vi "选择某框-子界面.vi"() -> ()   [LabVIEW 2018]
uses:
  <vilib>/vision/NI_Vision_Development_Module.lvlib
  <vilib>/Utility/NIReport.llb/Report Type.ctl
  <vilib>/Utility/NIReport.llb/NI_ReportGenerationCore.lvlib
panel:
  out "框组":T1(array[cluster])
  out "框号":dbl format="%#_13g"
  out "选中框灰度表":u32[](graph)
  out "最小灰度值":sgl
  out "最大灰度值":sgl
  out "平均值":sgl
  out "标准差":sgl
  in  "条件1-面积判断":T3(array[cluster]) {"Measurement Parameter" items=["Area"]; "下限" format="%.2f"; "上限" format="%.2f"}
  out "显示结果":string caption="所选区域信息"
  out "Particle Measurements (Pixels)":dbl[][](array[numeric]) format="%.2f"
  in  "报告生成":bool
  out "检查文件路径是否正确":bool caption="文件或文件夹存在？"
  out "保存路径":path
  in  "产品序号":string
  in  "部位":string="位置1"
  in  "类型":string="类型1"
  in  "合格性":string="合格"
  in  "检验人":string
  out "模板路径":path
  in  "分隔符（'\\'代码显示）":string="\t"
  in  "格式字符串":string="%f"
  out "所选区域检测结果":string[][](table)
  in  "查看完毕":bool
  in  "Color":u32[](array[colorbox])=[3381759, 16776770, 16777225, 6618880]
  in  "Overlay Type":u16[](array[ring])=[2, 1, 3, 0] items=["Rectangle", "Numbers", "Points", "Lines"]
  in  "条件2-灰度阈值":cluster{"下限":sgl, "上限":sgl}={"下限"=128.0, "上限"=255.0} {"下限" min=0 max=255 step=1; "上限" min=0 max=255 step=1}
  in  "Tab Control":T4
  out "原图":T5(plugin-control) caption="Original Image"
  out "阈值处理":T5(plugin-control) caption="Threshold Image"
  out "面积筛选":T5(plugin-control) caption="Reject Border and Fill Holes"
  out "缺陷统计":T5(plugin-control) caption="Filter Out Non Circles and Overlay Particle Area"
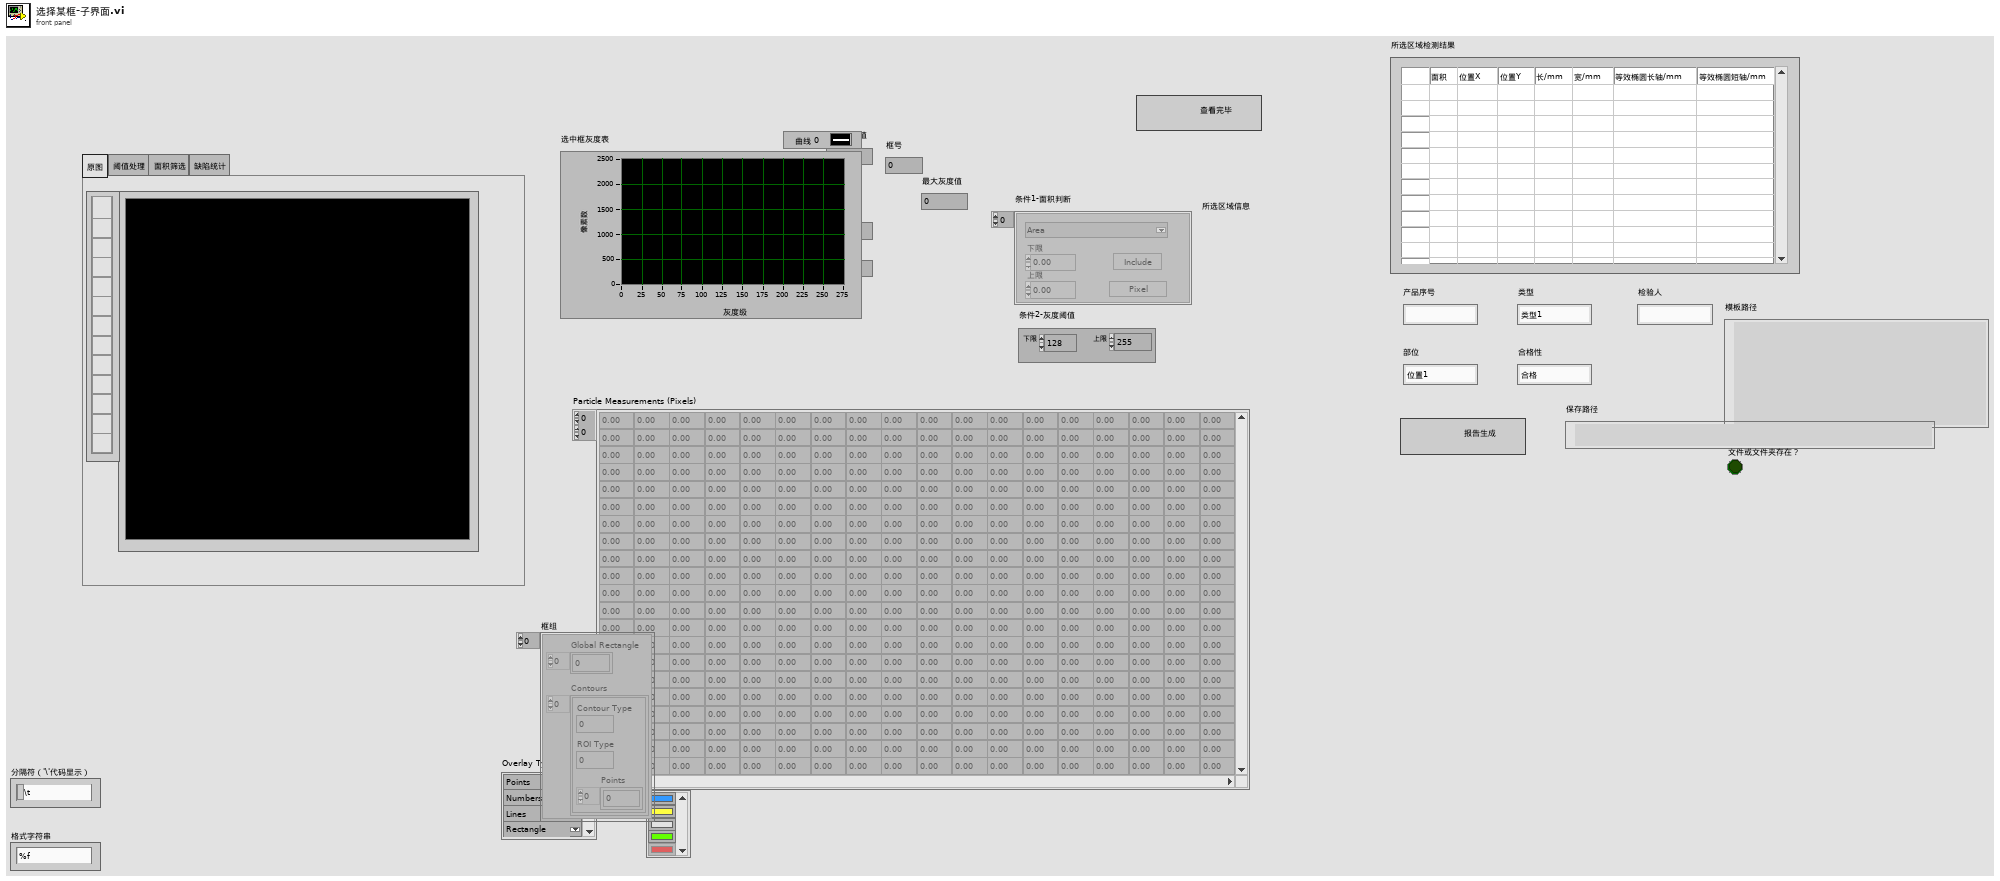
[diagram p1: front panel]
types:
  T1 = cluster{"Global Rectangle":i32[], "Contours":cluster{"Contour Type":u32, "ROI Type":u32, "Points":i32[]}[]}[]
  T2 = typedef "Particle Parameters" = i32
  T3 = cluster{"Measurement Parameter":T2, "下限":dbl, "上限":dbl, "Range":bool, "Measurement Type":bool}[]
  T4 = typedef "控件 1.ctl" = enum32{"原图", "阈值处理", "面积筛选", "缺陷统计"}
  T5 = typedef "IMAQ Image.ctl" = refnum<image>
  T6 = typedef "NI_ReportGenerationCore.lvlib/Report Type.ctl" = enum16{"HTML", "Word", "Excel"}
  T7 = cluster{"position (excel)":cluster{"row":i32, "column":i32}, "name (excel)":string, "bookmark (word)":string}
  T8 = typedef "Image Type" = u32
  T9 = cluster{"Global Rectangle":i32[], "Contours":cluster{"Contour Type":u32, "ROI Type":u32, "Points":i32[]}[]}
  T10 = typedef "IMAQ Rectangle" = cluster{"Left":i32, "Top":i32, "Right":i32, "Bottom":i32, "Rotation":dbl}
  T11 = cluster{"条件2-灰度阈值":cluster{"下限":sgl, "上限":sgl}, "Pixel Measurements":T2[], "Overlay Type":u16[], "Color":u32[]}
  T12 = cluster{"histogram":u32[], "Minimal Value":sgl, "Maximal Value":sgl, "Starting Value":sgl, "Interval Width":sgl, "Mean Value":sgl, "Standard  Variation":sgl, "Area (pixels)":i32}
  T13 = cluster{"Desired Font (Application)":enum16{"User-specified Font", "Application Font", "System Font", "Dialog Font"}, "[User-specified Font]":cluster{"Font Name":string, "Size":i16, "Strikeout?":bool, "Italic?":bool, "Underline?":bool, "Outline?":bool, "Shadow?":bool, "Bold?":bool, "Rotation Angle":dbl}, "Horizontal Alignment":i16, "Vertical Alignment":i16}
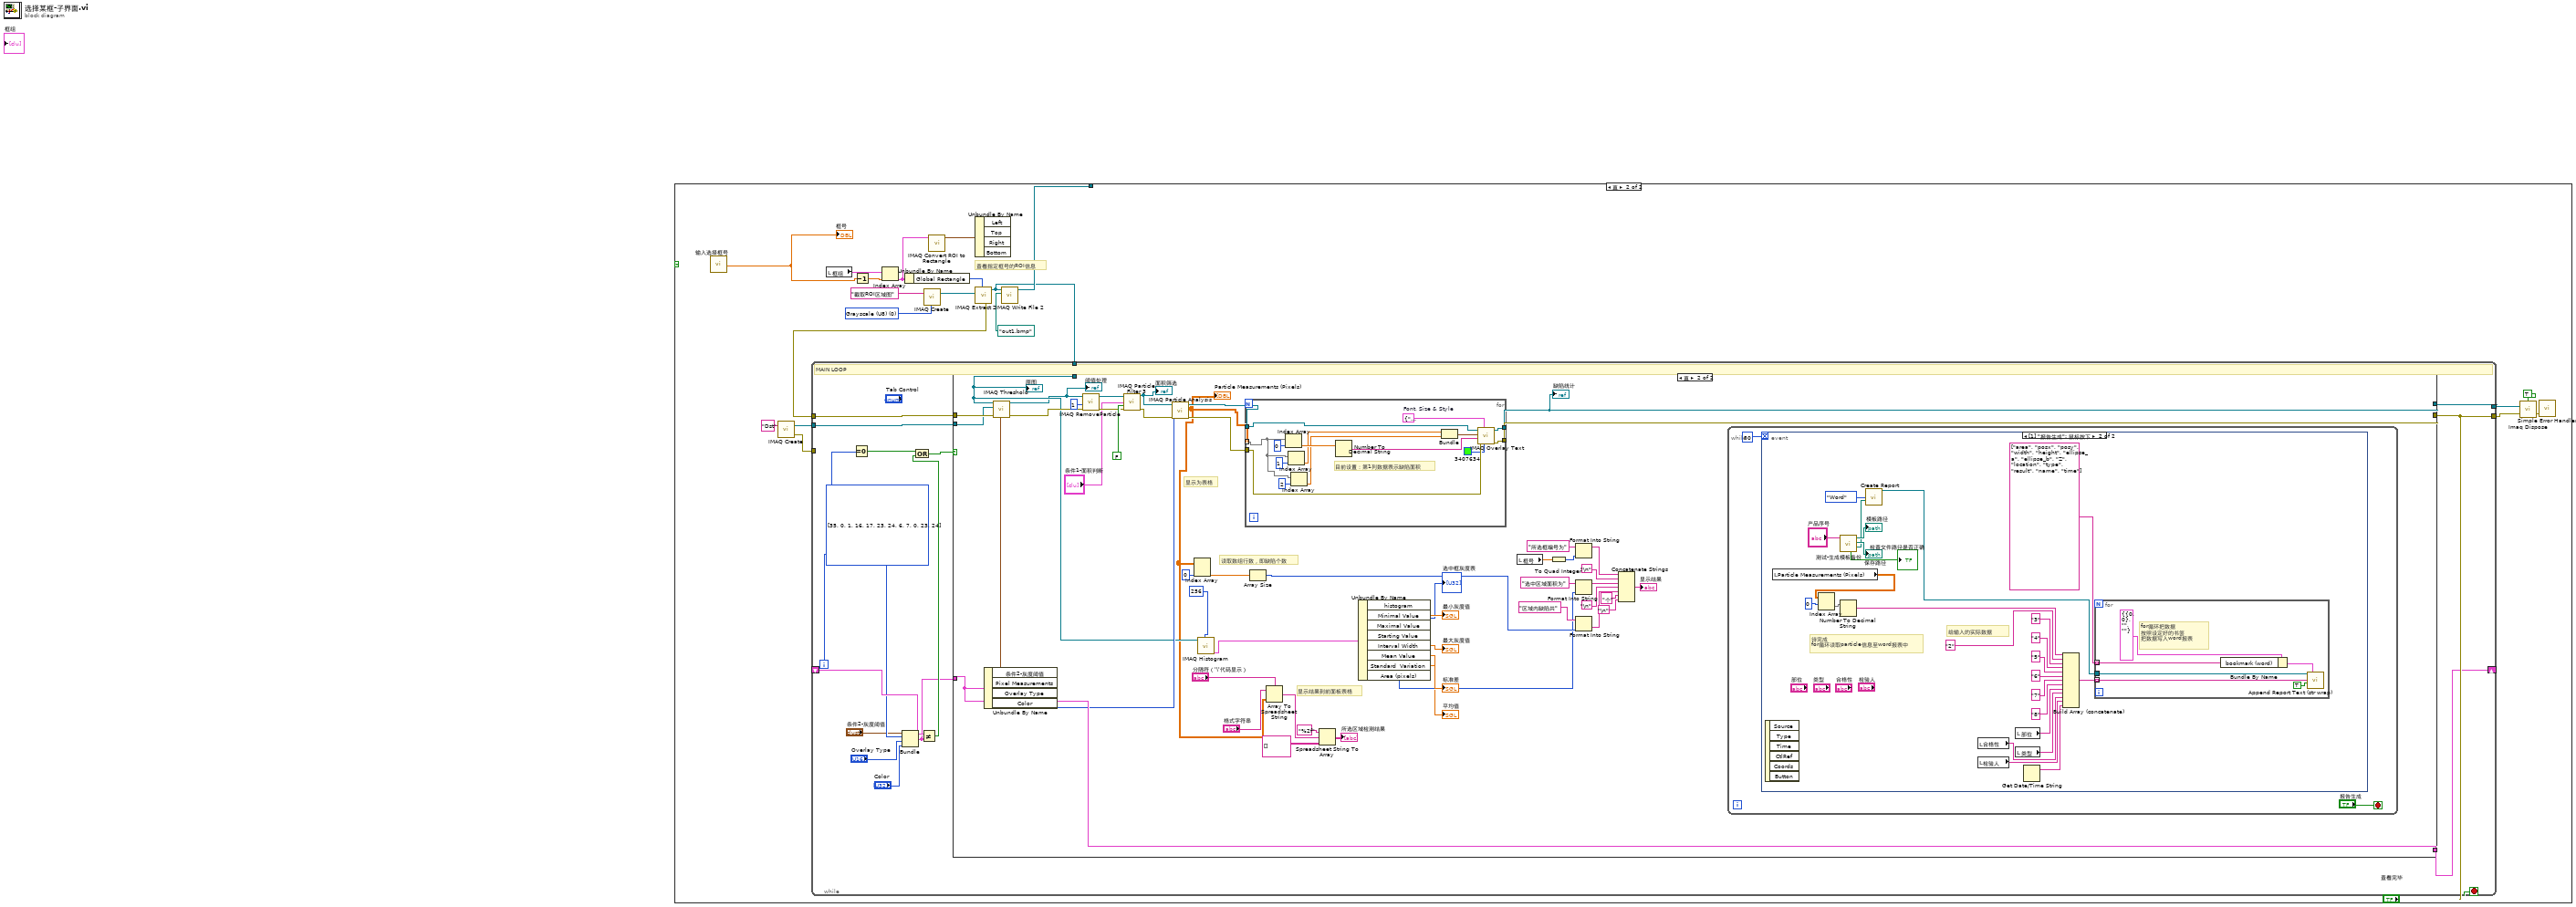
[diagram p0: block diagram]
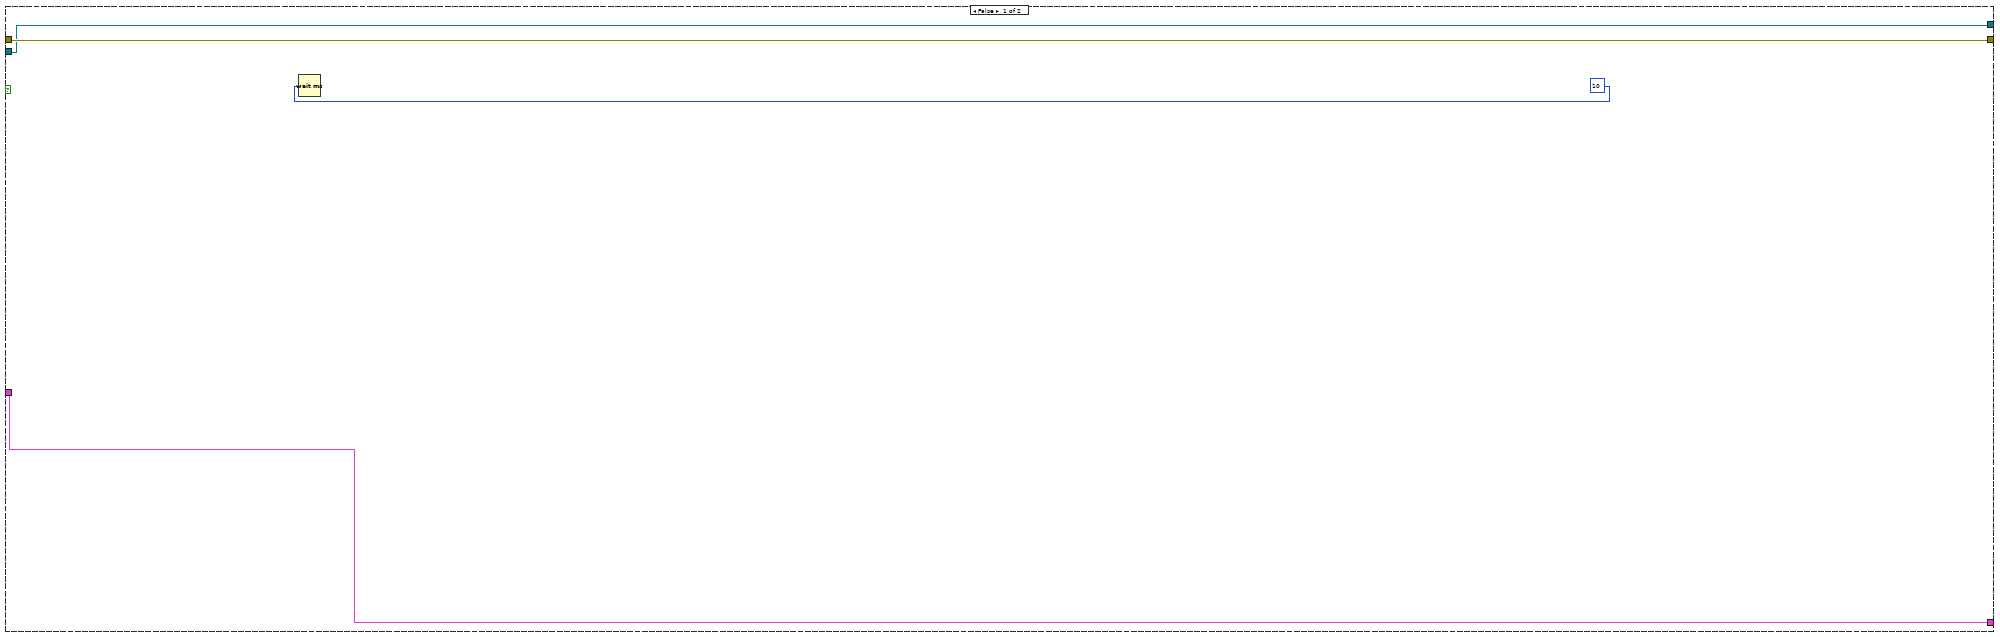
[diagram p3: hidden frame]
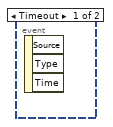
[diagram p4: hidden frame]
diagram:
  n1 = case shown="真" {
    selector: _ -> [_ _]
    tunnel: _ -> [_ w13]
    frame False {
      # "用户取消操作"
    }
    frame True {
      w17 = T8 0 items=["Grayscale (U8)", "Grayscale (I16)", "Grayscale (SGL)", "Complex (CSG)", "RGB (U32)", "HSL (U32)", "RGB (U64)", "Grayscale (U16)"] ("Image Type")
      # "查看指定框号的ROI信息"
      n2 = call "输入选择框号"() -> ("框号"=w1:dbl)  [unwired: 17 in, 2 out]
      "框号" <- w1
      n3 = call "IMAQ Create"("Image Name"="Dst") -> ("New Image"=w6:T5, "error out"=w5:errorcluster)  [unwired: 4 in]
      n4 = local read "框组"() -> (w19:T1)
      n5 = Decrement(x=w1) -> (x-1=w20:dbl)
      n6 = Index Array(array=w19, index=w20) -> (element=w12:T9)
      n7 = Unbundle By Name(w12) -> ("Global Rectangle"=w18:i32[])
      n8 = call "IMAQ Create"("Image Name"="截取ROI区域图", "Image Type"=w17) -> ("New Image"=w15:T5)  [unwired: 3 in, 1 out]
      n9 = call "IMAQ Convert ROI to Rectangle"("ROI Descriptor"=w12) -> ("Rectangle"=w14:T10)  [unwired: 8 in, 1 out]
      n10 = Unbundle By Name(w14) -> ()  [unwired: 4 out]
      n11 = call "IMAQ Extract 2"("Optional Rectangle"=w18, "Image Dst"=w15, "Image Src"=w13) -> ("error out"=w3:errorcluster, "Image Dst Out"=w2:T5)  [unwired: 7 in]
      n12 = while "MAIN LOOP" {
        tunnel: w3 -> [w28]
        tunnel: [w37] -> w10
        shift-right: [w34] -> _
        shift-left: _ -> [w32]
        tunnel: w6 -> [w29]
        tunnel: w5 -> [_]
        tunnel: [w27] -> w4
        tunnel: w2 -> [w24]
        i -> [w36]
        stop <- w38 stop-if-true
        w26 = T2[] [35, 0, 1, 16, 17, 23, 24, 6, 7, 0, 23, 24] items=["Center of Mass X", "Center of Mass Y", "First Pixel X", "First Pixel Y", "Bounding Rect Left", "Bounding Rect Top", "Bounding Rect Right", "Bounding Rect Bottom", "Max Feret Diameter Start X", "Max Feret Diameter Start Y", "Max Feret Diameter End X", "Max Feret Diameter End Y", "Max Horiz. Segment Length Left", "Max Horiz. Segment Length Right", "Max Horiz. Segment Length Row", "-", "Bounding Rect Width", "Bounding Rect Height", "Bounding Rect Diagonal", "Perimeter", "Convex Hull Perimeter", "Holes' Perimeter", "Max Feret Diameter", "Equivalent Ellipse Major Axis", "Equivalent Ellipse Minor Axis", "Equivalent Ellipse Minor Axis (Feret)", "Equivalent Rect Long Side", "Equivalent Rect Short Side", "Equivalent Rect Diagonal", "Equivalent Rect Short Side (Feret)", "Average Horiz. Segment Length", "Average Vert. Segment Length", "Hydraulic Radius", "Waddel Disk Diameter", "-", "Area", "Holes' Area", "Particle & Holes' Area", "Convex Hull Area", "Image Area", "-", "Number of Holes", "Number of Horiz. Segments", "Number of Vert. Segments", "-", "Orientation", "Max Feret Diameter Orientation", "-", "% Area/Image Area", "% Area/(Particle & Holes' Area)", "Ratio of Equivalent Ellipse Axes", "Ratio of Equivalent Rect Sides", "-", "Elongation Factor", "Compactness Factor", "Heywood Circularity Factor", "Type Factor", "-", "Sum X", "Sum Y", "Sum XX", "Sum XY", "Sum YY", "Sum XXX", "Sum XXY", "Sum XYY", "Sum YYY", "-", "Moment of Inertia XX", "Moment of Inertia XY", "Moment of Inertia YY", "Moment of Inertia XXX", "Moment of Inertia XXY", "Moment of Inertia XYY", "Moment of Inertia YYY", "Norm. Moment of Inertia XX", "Norm. Moment of Inertia XY", "Norm. Moment of Inertia YY", "Norm. Moment of Inertia XXX", "Norm. Moment of Inertia XXY", "Norm. Moment of Inertia XYY", "Norm. Moment of Inertia YYY", "Hu Moment 1", "Hu Moment 2", "Hu Moment 3", "Hu Moment 4", "Hu Moment 5", "Hu Moment 6", "Hu Moment 7"] ("Pixel Measurements")
        # "MAIN LOOP"
        n13 = Equal To 0?(x=w36) -> (x = 0?=w33:bool)
        n14 = Bundle("条件2-灰度阈值"="条件2-灰度阈值", "Pixel Measurements"=w26, "Overlay Type"="Overlay Type", "Color"="Color") -> (w30:T11)  [unwired: 1 in]
        n15 = Not Equal?(x=w32, y=w30) -> (x != y?=w31:bool)
        n16 = Compound Arithmetic op=OR(w33, w31) -> (w35:bool)
        n17 = case shown="真" w35 {
          tunnel: w28 -> [w42 w92]
          tunnel: [w39 w53] -> w27
          tunnel: [w42 w82] -> w37
          tunnel: [w41 w81] -> w34
          tunnel: w30 -> [w41 w81]
          tunnel: w29 -> [w39 w91]
          tunnel: w24 -> [_ w56]
          frame False {
            n18 = Wait (ms)(milliseconds to wait=u32 10) -> ()  [unwired: 1 out]
          }
          frame True {
            # "显示结果到前面板表格"
            # "读取数组行数，即缺陷个数"
            # "显示为表格"
            n19 = Unbundle By Name(w81) -> ("条件2-灰度阈值"=w80:cluster{"下限":sgl, "上限":sgl}, "Pixel Measurements"=w79:T2[])  [unwired: 2 out]
            n20 = call "IMAQ Threshold"("error in (no error)"=w92, "Range"=w80, "Image Dst"=w91, "Image Src"=w56) -> ("error out"=w87:errorcluster, "Image Dst Out"=w55:T5)  [unwired: 2 in, 4 out]
            "阈值处理" <- w55
            n21 = call "IMAQ RemoveParticle"("error in (no error)"=w87, "Number of Erosion"=1, "Image Src"=w55) -> ("error out"=w86:errorcluster, "Image Dst Out"=w89:T5)  [unwired: 7 in]
            n22 = call "IMAQ Particle Filter 3"("Image Src"=w89, "Selection Values"="条件1-面积判断", "Keep/Remove Particles (F)"=FALSE, "error in (no error)"=w86) -> ("Image Dst Out"=w54:T5, "error out"=w85:errorcluster)  [unwired: 9 in, 1 out]
            "面积筛选" <- w54
            n23 = call "IMAQ Particle Analysis"("error in (no error)"=w85, "Pixel Measurements"=w79, "Image"=w54) -> ("error out"=w83:errorcluster, "Particle Measurements (Pixels)"=w47:dbl[][], "Image Out (duplicate)"=w84:T5)  [unwired: 3 in, 3 out]
            "Particle Measurements (Pixels)" <- w47
            n24 = Index Array(array=w47, index (col)=0 ("禁用的索引 (列)")) -> (element=w50:dbl[])  [unwired: 1 in]
            n25 = call "IMAQ Histogram"("Number of Classes"=256, "Image"=w56) -> ("Histogram Report"=w59:T12)  [unwired: 8 in, 1 out]
            n26 = for {
              tunnel: w83 -> [w140]
              tunnel: [w139] -> w82
              tunnel: [w138] -> w53
              tunnel: w84 -> [w136]
              tunnel: w47 -> [w128] mode=indexing
              w135 = T13 {"Desired Font (Application)"=enum."Application Font", "[User-specified Font]"={"Font Name"="", "Size"=12, "Strikeout?"=FALSE, "Italic?"=FALSE, "Underline?"=FALSE, "Outline?"=FALSE, "Shadow?"=FALSE, "Bold?"=FALSE, "Rotation Angle"=0.0}, "Horizontal Alignment"=0, "Vertical Alignment"=0}  # Font, Size & Style
              # "目前设置：第1列数据表示缺陷面积"
              n27 = Index Array(array=w128, index=0 ("索引")) -> (element=w133:dbl)
              n28 = Index Array(array=w128, index=1 ("索引")) -> (element=w130:dbl)
              n29 = Index Array(array=w128, index=2 ("索引")) -> (element=w127:dbl)
              n30 = Number To Decimal String(number=w133) -> (decimal integer string=w134:string)  [unwired: 1 in]
              n31 = Bundle("Numeric"=w130, "Numeric"=w127) -> (w126:cluster{"Numeric":dbl, "Numeric":dbl})  [unwired: 1 in]
              n32 = call "IMAQ Overlay Text"("Text Color (black)"=u32 3407634, "Font, Size & Style"=w135, "error in (no error)"=w140, "String"=w134, "Origin"=w126, "Image"=w136) -> ("error out"=w139:errorcluster, "Image Out"=w138:T5)  [unwired: 4 in]
            }
            "缺陷统计" <- w53
            n33 = Array Size(array=w50) -> (size(s)=w66:i32)
            n34 = Array To Spreadsheet String(delimiter (Tab)="分隔符（'\\'代码显示）", array=w47, 3:"格式字符串") -> (spreadsheet string=w43:string)
            n35 = Spreadsheet String To Array(format string="%2f", spreadsheet string=w43, array type (2D Dbl)=string[][] [] ("Array")) -> (array=→"所选区域检测结果":string[][])  [unwired: 1 in]
            n36 = Unbundle By Name(w59) -> ("histogram"=→"选中框灰度表":u32[], "Minimal Value"=→"最小灰度值":sgl, "Maximal Value"=→"最大灰度值":sgl, "Mean Value"=→"平均值":sgl, "Standard  Variation"=→"标准差":sgl, "Area (pixels)"=w57:i32)  [unwired: 2 out]
            n37 = local read "框号"() -> (w68:dbl)
            n38 = To Quad Integer(1:w68) -> (0:w67:i64)
            n39 = Format Into String(initial string="所选框编号为" ("初始字符串"), w67) -> (resulting string=w69:string)  [unwired: 2 in, 1 out]
            n40 = Format Into String(initial string="选中区域面积为" ("字符串"), w57) -> (resulting string=w76:string)  [unwired: 2 in, 1 out]
            n41 = Format Into String(initial string="区域内缺陷共" ("初始字符串"), w66) -> (resulting string=w74:string)  [unwired: 2 in, 1 out]
            n42 = Concatenate Strings(w69, "\n", w76, "\n", w74, "个" ("字符串"), "\n") -> (→"显示结果":string)
            n43 = while {
              stop <- "报告生成" stop-if-true
              n44 = event shown="[1] \"报告生成\": 鼠标按下" {
                selector: _ -> [_ _]
                dyn-events: _ -> [_ _]
                timeout: 50 -> [_ _]
                event Timeout {
                  n45 = event-data() -> ()  [unwired: 1 in, 3 out]
                }
                event "报告生成": Mouse Down {
                  # "给输入的实际数据"
                  # "待完成\nfor循环读取particle信息至word报表中"
                  n46 = event-data() -> ()  [unwired: 1 in, 6 out]
                  n47 = local read "Particle Measurements (Pixels)"() -> (w96:dbl[][])
                  n48 = Index Array(array=w96, index (row)=0 ("索引 (行)")) -> (element=w99:dbl[])  [unwired: 1 in]
                  n49 = call "测试-生成模板备份.vi"("输入产品序号"="产品序号") -> ("new path"=w114:path, "保存路径"=→"保存路径":path, "模板路径"=→"模板路径":path, "检查文件路径是否正确"=→"检查文件路径是否正确":bool)  [unwired: 7 in]
                  n50 = Number To Decimal String(number=w99) -> (decimal integer string=w104:string[])  [unwired: 1 in]
                  n51 = call "Create Report.vi"("report type"=Report_Type."Word", "template (empty)"=w114) -> ("report out"=w95:refnum<class "NI_report.lvclass">)  [unwired: 12 in, 1 out]
                  n52 = local read "合格性"() -> (w101:string)
                  n53 = local read "检验人"() -> (w100:string)
                  n54 = local read "部位"() -> (w103:string)
                  n55 = local read "类型"() -> (w102:string)
                  n56 = Get Date/Time String() -> (date string=w106:string)  [unwired: 3 in, 1 out]
                  n57 = Build Array (concatenate)(w104, "2", "3", "4", "5" ("元素"), "6" ("元素"), "7" ("元素"), "8" ("元素"), w103, w102, w101, w100, w106) -> (w97:string[])
                  n58 = for {
                    tunnel: w95 -> [w122]
                    tunnel: string[] ["area", "posx", "posy", "width", "height", "ellipse_a", "ellipse_b", "Z", "location", "type", "result", "name", "time"] -> [w121] mode=indexing
                    tunnel: w97 -> [w120] mode=indexing
                    # "for循环把数据\n按照设定好的书签 \n把数据写入word报表"
                    n59 = Bundle By Name(cluster=T7 {"position (excel)"={"row"=0, "column"=0}, "name (excel)"="", "bookmark (word)"=""} ("MS Office parameters"), "bookmark (word)"=w121) -> (w125:T7)
                    n60 = call "Append Report Text (str wrap).vi"("report in"=w122, "MS Office parameters"=w125, "text"=w120, "append on new line? (F)"=TRUE) -> ()  [unwired: 8 in, 4 out]
                  }
                }
              }
            }
            "原图" <- w56
          }
        }
        n61 = Or(x=w37, y="查看完毕") -> (x .or. y?=w38:bool)
      }
      n62 = call-poly "IMAQ Write File 2"("File Path"=path "out1.bmp", "Image"=w2) -> ()  [unwired: 8 in, 2 out]
      n63 = call "Imaq Dispose"("All Images? (No)"=TRUE, "Image"=w4, "error in (no error)"=w10) -> ("error out"=w9:errorcluster)  [unwired: 3 in]
      n64 = call <vilib>:"Simple Error Handler.vi"("error in (no error)"=w9) -> ()  [unwired: 4 in, 5 out]
    }
  }
